vi "Pressure to Caller.vi"(8 "error in (no error)":errorcluster, 10 "Analog Input Waveform":waveform(dbl), 11 "APG in":refnum<class "APG.lvclass">) -> (0 "error out":errorcluster)   [LabVIEW 2021, in "APG.lvclass"]
uses:
  APG.lvclass
  APG.lvclass/APG.ctl
  <vilib>/ActorFramework/Actor/Actor.lvclass
  Pressure Gauges/Pressure Gauges Messages/Received Pressure Msg/Received Pressure Msg.lvclass
  C:/Program Files/National Instruments/LabVIEW 2021/vi.lib/MGI/Panel Manager/Panel Actor/Panel Actor/Panel Actor.lvclass
  C:/Program Files/National Instruments/LabVIEW 2021/vi.lib/ActorFramework/Actor/Actor.lvclass
  C:/git/Pressure-Gauges/Source/APG/APG/APG.lvclass
  C:/Program Files/National Instruments/LabVIEW 2021/vi.lib/NathanCo/Analog Tasks/Analog Input/Analog Input Interface Messages/Analog Input Interface Messages/Analog Input Interface Messages.lvclass
  C:/git/Pressure-Gauges/Source/Pressure to Caller/Pressure to Caller.lvclass
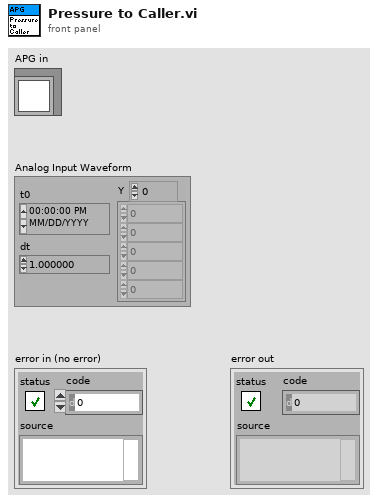
[diagram p1: front panel]
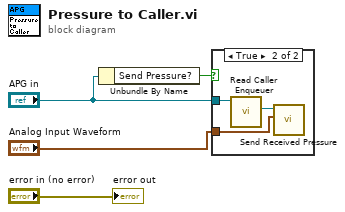
[diagram p0: block diagram]
diagram:
  n1 = Unbundle By Name("APG in") -> ("Send Pressure?"=w3:bool)
  n2 = case shown="True" w3 {
    tunnel: "APG in" -> [_ w7]
    tunnel: "Analog Input Waveform" -> [_ w5]
    frame False {
    }
    frame True {
      n3 = call <vilib>:"Read Caller Enqueuer.vi"("Actor"=w7) -> ("Caller Enqueuer"=w6:refnum<class "Message Enqueuer.lvclass">)  [unwired: 10 in]
      n4 = call "Send Received Pressure.vi"("Received Pressure"=w5, "Message Enqueuer"=w6) -> ()  [unwired: 8 in, 2 out]
    }
  }
  "error out" <- "error in (no error)"
